vi "Register Subsystem.vi"(8 "error in (no error)":errorcluster, 9 "Subsystem Name (optional)":string, 10 "JKI SMO in":refnum<class "SMO.lvclass">) -> (0 "error out":errorcluster, 1 "Attribute.Identity":refnum<class "Attribute.Identity.lvclass">, 2 "JKI SMO out":refnum<class "SMO.lvclass">)   [LabVIEW 2019, in "Registry-SMO.lvclass"]
doc: "JKI State Machine Objects (SMO) 1.3.0.56\nJKI - JKI\nCopyright (c) 2017, JKI"
uses:
  Registry-SMO.lvclass
  SMO/SMO.lvclass
  Support/Attribute.Identity/Attribute.Identity.lvclass
  SMO_Info--Cluster.ctl
  Registry-SMO.lvclass/Registry-SMO.ctl
  Support/Attribute.Identity/Attribute.Identity.lvclass/Attribute.Identity.ctl
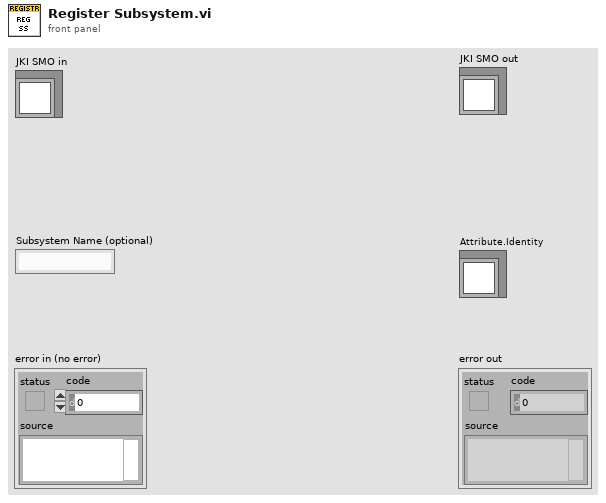
[diagram p1: front panel]
types:
  T1 = typedef "Registry-SMO.lvclass/SMO_Info--Cluster.ctl" = cluster{"Name":string, "Shared Resource":bool}
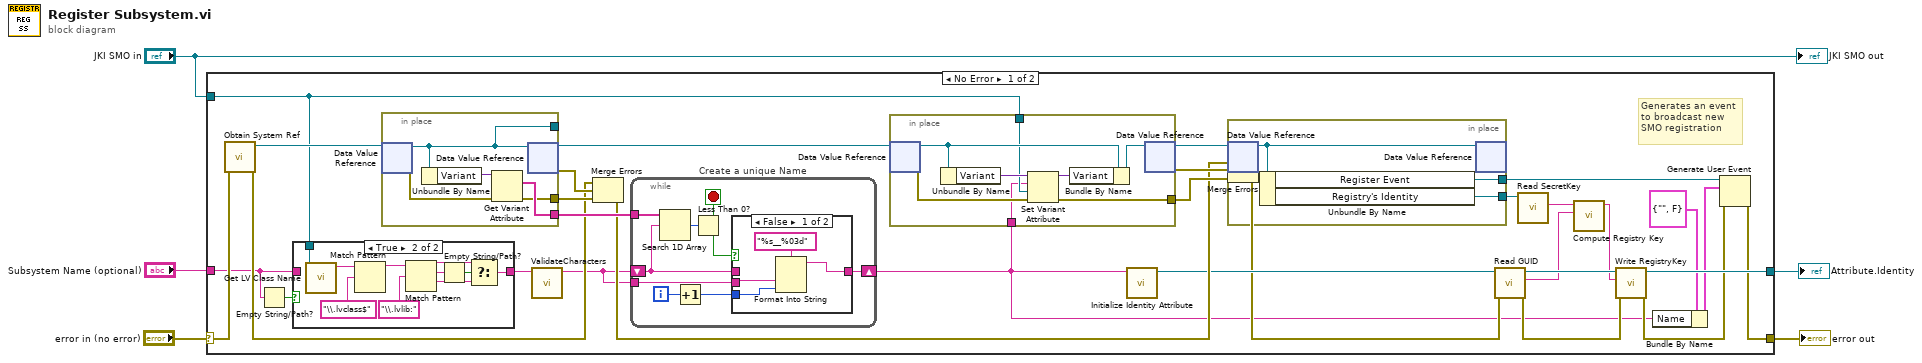
[diagram p0: block diagram]
diagram:
  n1 = case shown="No Error" "error in (no error)" {
    selector: "error in (no error)" -> [w34 w77]
    tunnel: [w11 w77] -> w4
    tunnel: "Subsystem Name (optional)" -> [w9 _]
    tunnel: "JKI SMO in" -> [w6 _]
    tunnel: [w24 _] -> w2
    frame No Error {
      # "Generates an event\nto broadcast new\nSMO registration"
      n2 = call "Obtain System Ref.vi"("error in (no error)"=w34) -> ("error out"=w27:errorcluster, "JKI SMO System"=w33:refnum<data-value>)  [unwired: 9 in]
      n3 = Empty String/Path?(string/path=w9) -> (empty?=w32:bool)
      n4 = case shown="True" w32 {
        tunnel: w9 -> [w53 _]
        tunnel: [w53 w54] -> w8
        tunnel: w6 -> [_ w63]
        frame False {
        }
        frame True {
          n5 = call <vilib>:"Get LV Class Name.vi"("object"=w63) -> ("class name"=w55:string)  [unwired: 9 in, 1 out]
          n6 = Match Pattern(string=w55, regular expression="\\.lvclass$") -> (before substring=w61:string)  [unwired: 1 in, 3 out]
          n7 = Match Pattern(string=w61, regular expression="\\.lvlib:") -> (before substring=w57:string, match substring=w59:string, after substring=w56:string)  [unwired: 1 in, 1 out]
          n8 = Empty String/Path?(string/path=w59) -> (empty?=w58:bool)
          n9 = Select(t=w57, s=w58, f=w56) -> (s? t:f=w54:string)
        }
      }
      n10 = in-place {
        in-place-border: [w66] -> w31
        in-place-border: [w65] -> w28
        in-place-border: [w64] -> _
        n11 = in-place-dvr #1(w33) -> (w64:refnum<class "Registry-SMO.lvclass">, w67:errorcluster)
        n12 = Unbundle By Name(w64) -> ("Variant"=w68:variant)
        n13 = Get Variant Attribute(Variant=w68, error in=w67) -> (names=w66:string[], error out=w65:errorcluster)  [unwired: 2 in, 2 out]
        n14 = in-place-dvr #1(w64) -> (w30:refnum<data-value>, w29:errorcluster)
      }
      n15 = call "ValidateCharacters.vi"("Subsystem Name (optional)"=w8) -> ("Validated characters"=w7:string)  [unwired: 10 in]
      n16 = Merge Errors(w27, w29, w28) -> (w26:errorcluster)
      n17 = while "Create a unique Name" {
        tunnel: w31 -> [w47]
        shift-right: [w43] -> w10
        shift-left: w7 -> [w44]
        tunnel: w7 -> [w42]
        i -> [w41]
        stop <- w45 stop-if-true
        n18 = Search 1D Array(1D array=w47, element=w44) -> (index of element=w46:i32)  [unwired: 1 in]
        n19 = Increment(x=w41) -> (x+1=w40:i32)
        n20 = Less Than 0?(x=w46) -> (x < 0?=w45:bool)
        n21 = case shown="False" w45 {
          tunnel: w44 -> [_ w52]
          tunnel: [w50 w52] -> w43
          tunnel: w42 -> [w51 _]
          tunnel: w40 -> [w49 _]
          frame False {
            n22 = Format Into String(format string="%s__%03d", w51, w49) -> (resulting string=w50:string)  [unwired: 2 in, 1 out]
          }
          frame True {
            # "Name is unique"
          }
        }
      }
      n23 = in-place {
        in-place-border: w6 -> [w73]
        in-place-border: [w71] -> w35
        in-place-border: w10 -> [w69]
        n24 = in-place-dvr #2(w30) -> (w76:refnum<class "Registry-SMO.lvclass">, w70:errorcluster)
        n25 = Unbundle By Name(w76) -> ("Variant"=w74:variant)
        n26 = Set Variant Attribute(Variant=w74, name=w69, value=w73, error in=w70) -> (Variant out=w72:variant, error out=w71:errorcluster)  [unwired: 1 out]
        n27 = Bundle By Name(cluster=w76, "Variant"=w72) -> (w75:refnum<class "Registry-SMO.lvclass">)
        n28 = in-place-dvr #2(w75) -> (w25:refnum<data-value>, w36:errorcluster)
      }
      n29 = call "Initialize Identity Attribute.vi"("Name"=w10) -> ("Attribute.Identity"=w23:refnum<class "Attribute.Identity.lvclass">)  [unwired: 10 in]
      n30 = in-place {
        in-place-border: [w38] -> w21
        in-place-border: [w37] -> w15
        n31 = in-place-dvr #3(w25) -> (w39:refnum<class "Registry-SMO.lvclass">)  [unwired: 1 out]
        n32 = Unbundle By Name(w39) -> ("Register Event"=w37:refnum<user-event>, "Registry's Identity"=w38:refnum<class "Attribute.Identity.lvclass">)
        n33 = in-place-dvr #3(w39) -> ()  [unwired: 2 out]
      }
      n34 = Merge Errors(w26, w36, w35) -> (w17:errorcluster)
      n35 = call "Read GUID.vi"("error in (no error)"=w17, "Attribute.Identity in"=w23) -> ("error out"=w16:errorcluster, "GUID"=w19:string, "Attribute.Identity out"=w22:refnum<class "Attribute.Identity.lvclass">)  [unwired: 7 in]
      n36 = call "Read SecretKey.vi"("Attribute.Identity in"=w21) -> ("SecretKey"=w20:string)  [unwired: 8 in, 2 out]
      n37 = call "Compute Registry Key.vi"("SMO GUID"=w19, "Registry's SecretKey"=w20) -> ("Registry Key"=w18:string)  [unwired: 9 in]
      n38 = call "Write RegistryKey.vi"("error in (no error)"=w16, "RegistryKey"=w18, "Attribute.Identity in"=w22) -> ("error out"=w12:errorcluster, "Attribute.Identity out"=w24:refnum<class "Attribute.Identity.lvclass">)  [unwired: 7 in]
      n39 = Bundle By Name(cluster=T1 {"Name"="", "Shared Resource"=FALSE} ("Cluster"), "Name"=w10) -> (w13:T1)
      n40 = Generate User Event(user event=w15, event data cluster=w13, error in=w12) -> (error out=w11:errorcluster)  [unwired: 1 in, 1 out]
    }
    frame Error {
    }
  }
  "error out" <- w4
  "Attribute.Identity" <- w2
  "JKI SMO out" <- "JKI SMO in"
